vi "Get Named Range Values (String).vi"(8 "error in":errorcluster, 9 "Sheet Name":string, 10 "Named Range Identifier":string, 11 "SpreadsheetDocument":refnum<k24>) -> (0 "error out":errorcluster, 2 "Cells":string[][](array[string]), 3 "SpreadsheetDocument out":refnum<k24>)   [LabVIEW 2019, in "Open Xml.lvlib"]
uses:
  Open Xml.lvlib
  D:/git/Open-Xml-LabVIEW/Source/DocumentFormat.OpenXml.dll
  DocumentFormat.OpenXml.dll
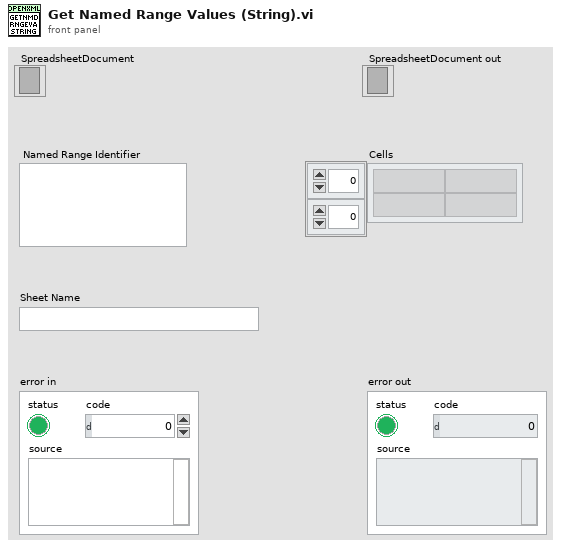
[diagram p1: front panel]
types:
  T1 = cluster{"Number":dbl, "String":string, "Boolean":bool, "Time Stamp":timestamp, "Error":errorcluster}[][]
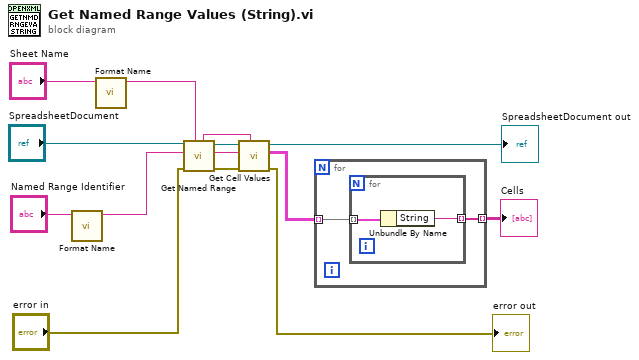
[diagram p0: block diagram]
diagram:
  n1 = call "Format Name.vi"("Sheet Name"="Named Range Identifier") -> ("Formatted Sheet Name"=w2:string)  [unwired: 10 in]
  n2 = call "Format Name.vi"("Sheet Name"="Sheet Name") -> ("Formatted Sheet Name"=w1:string)  [unwired: 10 in]
  n3 = call "Get Named Range.vi"("Sheet Name"=w1, "error in"="error in", "Range Identifier"=w2, "SpreadsheetDoc in"="SpreadsheetDocument") -> ("error out"=w7:errorcluster, "Range"=w11:string, "SpreadsheetDoc out"=w10:refnum<k24>, "Sheet Name"=w8:string)  [unwired: 4 in]
  n4 = call "Get Cell Values.vi"("Sheet Name"=w8, "error in"=w7, "Cell Addresses"=w11, "SpreadsheetDoc in"=w10) -> ("error out"=→"error out":errorcluster, "Cell Values"=w6:T1, "SpreadsheetDoc out"=→"SpreadsheetDocument out":refnum<k24>)  [unwired: 4 in, 1 out]
  n5 = for {
    tunnel: w6 -> [w16] mode=indexing
    tunnel: [w15] -> w5 mode=indexing
    n6 = for {
      tunnel: w16 -> [w18] mode=indexing
      tunnel: [w17] -> w15 mode=indexing
      n7 = Unbundle By Name(w18) -> ("String"=w17:string)
    }
  }
  "Cells" <- w5
